vi "zadanie_1.vi"() -> ()   [LabVIEW 2020]
panel:
  in  "Enum":T1(ring)
  in  "?":bool
  out "wynik":dbl
  in  "liczba B":dbl
  in  "liczba A":dbl
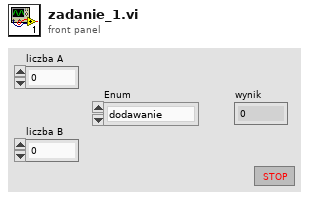
[diagram p1: front panel]
types:
  T1 = enum16{"dodawanie", "odejmowanie", "mnożenie", "dzielenie"}
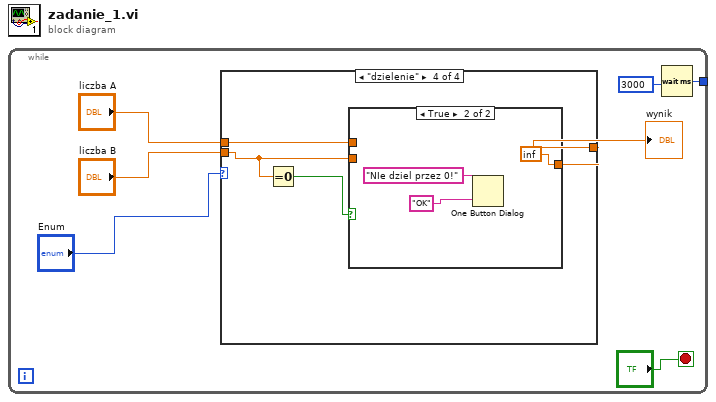
[diagram p0: block diagram]
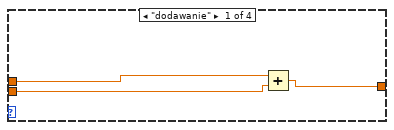
[diagram p2: hidden frame]
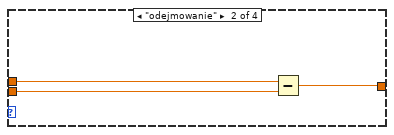
[diagram p3: hidden frame]
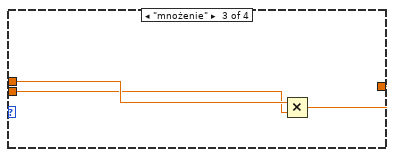
[diagram p4: hidden frame]
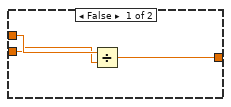
[diagram p5: hidden frame]
diagram:
  n1 = while {
    tunnel: [w2] -> _
    stop <- "?" stop-if-true
    n2 = case shown="\"dzielenie\"" "Enum" {
      tunnel: "liczba A" -> [w10 w13 w16 w19]
      tunnel: "liczba B" -> [w9 w12 w15 w20]
      tunnel: [w8 w11 w14 w18] -> w5
      frame "dodawanie" {
        n3 = Add(x=w10, y=w9) -> (x+y=w8:dbl)
      }
      frame "odejmowanie" {
        n4 = Subtract(x=w13, y=w12) -> (x-y=w11:dbl)
      }
      frame "mnożenie" {
        n5 = Multiply(x=w16, y=w15) -> (x*y=w14:dbl)
      }
      frame "dzielenie" {
        n6 = Equal To 0?(x=w20) -> (x = 0?=w17:bool)
        n7 = case shown="True" w17 {
          tunnel: w20 -> [w22 _]
          tunnel: w19 -> [w23 _]
          tunnel: [w21 inf] -> w18
          frame False {
            n8 = Divide(x=w23, y=w22) -> (x/y=w21:dbl)
          }
          frame True {
            n9 = One Button Dialog(message="NIe dziel przez 0!", button name ("OK")="OK") -> ()  [unwired: 1 out]
          }
        }
      }
    }
    "wynik" <- w5
    n10 = Wait (ms)(milliseconds to wait=3000) -> (millisecond timer value=w2:u32)
  }
